vi "F Dwf Digital I2c Write Read.vi"(0 "hdwf":i32, 1 "rgRx":string, 2 "pNak":i32, 5 "adr8bits":u8, 7 "rgbTx":string, 9 "cTx":i32, 11 "error in (no error)":errorcluster, 12 "cRx":i32) -> (3 "rgRx out":string, 4 "pNak out":i32, 6 "function return":i32, 8 "rgbTx out":string, 15 "error out":errorcluster)   [LabVIEW 2021, in "Olasdwf.lvlib"]
doc: "DWFAPI int FDwfDigitalI2cWriteRead(HDWF hdwf, unsigned char adr8bits, unsigned char *rgbTx, int cTx, unsigned char *rgRx, int cRx, int *pNak);"
uses:
  Olasdwf.lvlib
  Windows/System32/dwf.dll
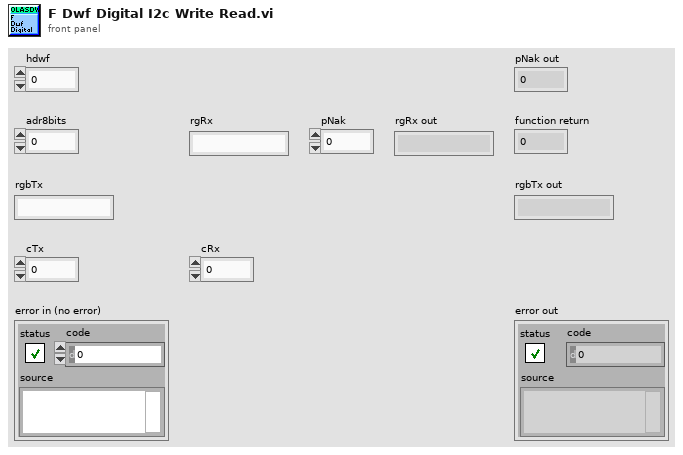
[diagram p1: front panel]
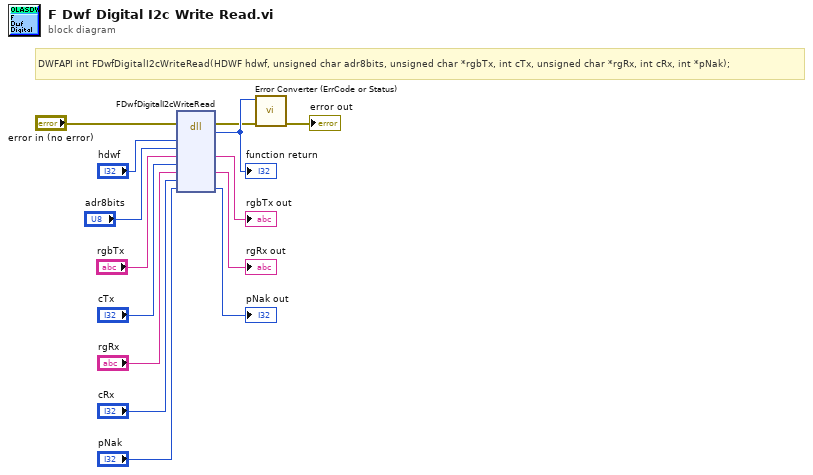
[diagram p0: block diagram]
diagram:
  # "DWFAPI int FDwfDigitalI2cWriteRead(HDWF hdwf, unsigned char adr8bits, unsigned char *rgbTx, int cTx, unsigned char *rgRx, int cRx, int *pNak);"
  n1 = dll-call lib="/Windows/System32/dwf.*" fn="FDwfDigitalI2cWriteRead"(error in="error in (no error)", "hdwf"="hdwf", "adr8bits"="adr8bits", "rgbTx"="rgbTx", "cTx"="cTx", "rgRx"="rgRx", "cRx"="cRx", "pNak"="pNak") -> (error out=w2:errorcluster, w14:i32, "rgbTx"=→"rgbTx out":string, "rgRx"=→"rgRx out":string, "pNak"=→"pNak out":i32)  [unwired: 6 in, 1 out]
  "function return" <- w14
  n2 = call "Error Converter (ErrCode or Status).vi"("error in (no error)"=w2, "error code"=w14) -> ("error out"=→"error out":errorcluster)  [unwired: 9 in]
